vi "TX OOB Test Cases.vi"() -> (0 "error out":errorcluster, 2 "status":string, 3 "pass":bool)   [LabVIEW 2021]
uses:
  <vilib>/CIF Foundation/CIF Out of Band Commands/CIFOutOfBand.lvclass/CIFOutOfBand.ctl
  OOB_Tx/Typedef/OOB Core Commands.ctl
  typedef/Channel List for OOB.ctl
  <vilib>/CIF Foundation/CIF Channels Core/CIFChannels/Typedef/Direction.ctl
  OOB_Tx/Typedef/FIFO Publisher Return.ctl
  OOB_Tx/Private/Command Settings.vi
  <vilib>/CIF Foundation/CIF Out of Band Commands/Accessors/Write Local OOB Data.vi
  <vilib>/CIF Foundation/CIF Out of Band Commands/Queue Command.vi
  <vilib>/CIF Foundation/CIF Out of Band Commands/Utilities/Command to Bitwise Command.vi
  <vilib>/CIF Foundation/CIF Out of Band Commands/Accessors/Read Local OOB Data.vi
  <vilib>/CIF Foundation/CIF Out of Band Commands/Read Commands.vi
  OOB_Tx/Private/Read Payload.vi
  OOB_Tx/ChnMngOOB_Tx.lvclass
  C:/Program Files/National Instruments/LabVIEW 2021/vi.lib/CIF Foundation/CIF Out of Band Commands/CIFOutOfBand.lvclass
  <vilib>/CIF Foundation/CIF Out of Band Commands/Init OOB.vi
  <vilib>/CIF Foundation/CIF Out of Band Commands/CIFOutOfBand.lvclass
  <vilib>/CIF Foundation/CIF Channels Core/CIFChannels/CIFChannels.lvclass
  CIFChannelMng.lvclass
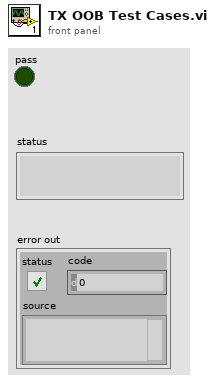
[diagram p1: front panel]
types:
  T1 = typedef "CIFChannelMng.lvclass/Channel List for OOB.ctl" = cluster{"Name":string, "Direction":T2, "Type":string, "Connected?":bool, "Connected Name":string, "Custom Config Data":u8[], "Forced?":bool}
  T2 = typedef "CIFChannels.lvclass/Direction.ctl" = enum16{"Publisher", "Subscriber"}
  T3 = typedef "ChnMngOOB_Tx.lvclass/OOB Core Commands.ctl" = enum8{"Channel List", "New FIFO Pub"}
  T4 = typedef "ChnMngOOB_Tx.lvclass/FIFO Publisher Return.ctl" = cluster{"FIFO Pub Name":string, "error":errorcluster, "Added":bool}
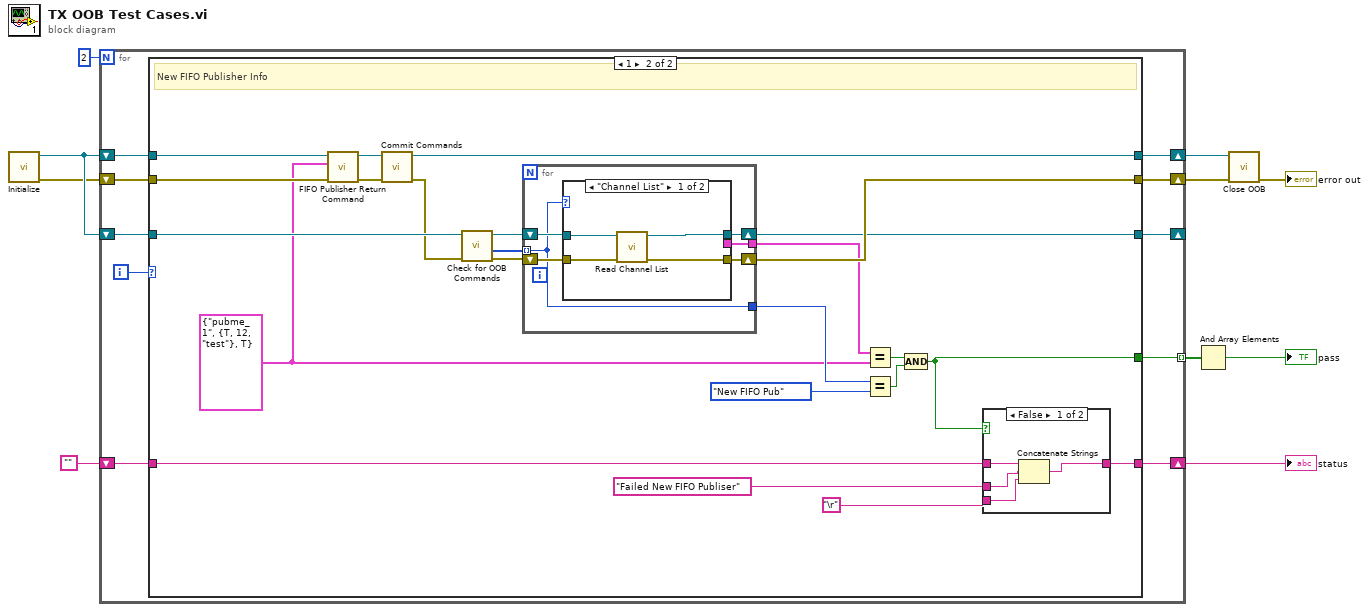
[diagram p0: block diagram]
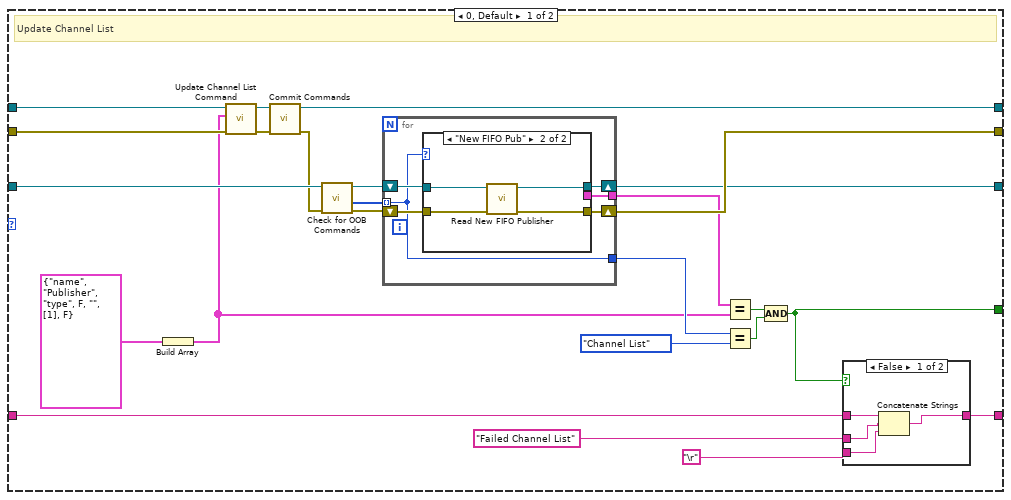
[diagram p2: hidden frame]
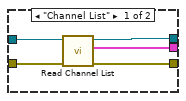
[diagram p3: hidden frame]
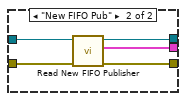
[diagram p5: hidden frame]
diagram:
  n1 = call "Initialize.vi"() -> ("error out"=w1:errorcluster, "CoreOOB_Tx out"=w2:refnum<class "ChnMngOOB_Tx.lvclass">)  [unwired: 10 in]
  n2 = for {
    N: 2 -> [_]
    tunnel: [w20] -> w8 mode=indexing
    shift-right: [w17] -> w9
    shift-left: w1 -> [w19]
    shift-right: [w12] -> w10
    shift-left: w2 -> [w18]
    shift-right: [w11] -> _
    shift-left: w2 -> [w15]
    shift-right: [w13] -> w5
    shift-left: "" -> [w14]
    i -> [w16]
    n3 = case shown="1" w16 {
      tunnel: [w36 w79] -> w20
      tunnel: w19 -> [w28 w70]
      tunnel: w18 -> [w29 w71]
      tunnel: [w44 w87] -> w17
      tunnel: [w21 w66] -> w12
      tunnel: w15 -> [w34 w77]
      tunnel: [w43 w86] -> w11
      tunnel: w14 -> [w42 w85]
      tunnel: [w41 w84] -> w13
      frame 0, Default {
        # "Update Channel List"
        n4 = Build Array(T1 {"Name"="name", "Direction"=enum."Publisher", "Type"="type", "Connected?"=FALSE, "Connected Name"="", "Custom Config Data"=[1], "Forced?"=FALSE} ("value")) -> (w25:T1[])
        n5 = call "Update Channel List Command.vi"("error in"=w28, "Channel List"=w25, "CoreOOB_Tx in"=w29) -> ("error out"=w23:errorcluster, "CoreOOB_Tx out"=w24:refnum<class "ChnMngOOB_Tx.lvclass">)  [unwired: 7 in]
        n6 = call <vilib>:"Commit Commands.vi"("error in"=w23, "OOB in"=w24) -> ("error out"=w22:errorcluster, "OOB out"=w21:refnum<class "ChnMngOOB_Tx.lvclass">)  [unwired: 8 in]
        n7 = call "Check for OOB Commands.vi"("error in (no error)"=w22, "CoreOOB_Tx in"=w34) -> ("error out"=w33:errorcluster, "Commands"=w31:T3[], "CoreOOB_Tx out"=w32:refnum<class "ChnMngOOB_Tx.lvclass">)  [unwired: 6 in, 1 out]
        n8 = for {
          tunnel: w31 -> [w46] mode=indexing
          shift-right: [w50] -> w44
          shift-left: w33 -> [w48]
          shift-right: [w49] -> w43
          shift-left: w32 -> [w47]
          tunnel: [w46] -> w35
          tunnel: [w45] -> w27
          n9 = case shown="\"New FIFO Pub\"" w46 {
            tunnel: w47 -> [w55 w59]
            tunnel: w48 -> [w54 w58]
            tunnel: [w53 w56] -> w49
            tunnel: [w52 w57] -> w50
            tunnel: [w51 _] -> w45
            frame "Channel List" {
              n10 = call "Read Channel List.vi"("error in"=w54, "CoreOOB_Tx in"=w55) -> ("error out"=w52:errorcluster, "Channel List"=w51:T1[], "CoreOOB_Tx out"=w53:refnum<class "ChnMngOOB_Tx.lvclass">)  [unwired: 7 in]
            }
            frame "New FIFO Pub" {
              n11 = call "Read New FIFO Publisher.vi"("error in"=w58, "CoreOOB_Tx in"=w59) -> ("error out"=w57:errorcluster, "CoreOOB_Tx out"=w56:refnum<class "ChnMngOOB_Tx.lvclass">)  [unwired: 7 in, 1 out]
            }
          }
        }
        n12 = Equal?(x=w27, y=w25) -> (x = y?=w38:bool)
        n13 = Equal?(x=w35, y=OOB_Core_Commands."Channel List") -> (x = y?=w37:bool)
        n14 = Compound Arithmetic op=AND(w38, w37) -> (w36:bool)
        n15 = case shown="False" w36 {
          tunnel: w42 -> [w63 w64]
          tunnel: [w60 w64] -> w41
          tunnel: "Failed Channel List" -> [w62 _]
          tunnel: "\r" -> [w61 _]
          frame False {
            n16 = Concatenate Strings(w63, w62, w61) -> (w60:string)
          }
          frame True {
          }
        }
      }
      frame 1 {
        w65 = T4 {"FIFO Pub Name"="pubme_1", "error"={"status"=TRUE, "code"=12, "source"="test"}, "Added"=TRUE} ("FIFO Publisher")
        # "New FIFO Publisher Info"
        n17 = call "FIFO Publisher Return Command.vi"("error in"=w70, "FIFO Publisher"=w65, "CoreOOB_Tx in"=w71) -> ("error out"=w68:errorcluster, "CoreOOB_Tx out"=w69:refnum<class "ChnMngOOB_Tx.lvclass">)  [unwired: 7 in]
        n18 = call <vilib>:"Commit Commands.vi"("error in"=w68, "OOB in"=w69) -> ("error out"=w67:errorcluster, "OOB out"=w66:refnum<class "ChnMngOOB_Tx.lvclass">)  [unwired: 8 in]
        n19 = call "Check for OOB Commands.vi"("error in (no error)"=w67, "CoreOOB_Tx in"=w77) -> ("error out"=w76:errorcluster, "Commands"=w74:T3[], "CoreOOB_Tx out"=w75:refnum<class "ChnMngOOB_Tx.lvclass">)  [unwired: 6 in, 1 out]
        n20 = for {
          tunnel: w74 -> [w89] mode=indexing
          shift-right: [w93] -> w87
          shift-left: w76 -> [w91]
          shift-right: [w92] -> w86
          shift-left: w75 -> [w90]
          tunnel: [w89] -> w78
          tunnel: [w88] -> w72
          n21 = case shown="\"Channel List\"" w89 {
            tunnel: w90 -> [w97 w102]
            tunnel: w91 -> [w96 w101]
            tunnel: [w95 w99] -> w92
            tunnel: [w94 w100] -> w93
            tunnel: [_ w98] -> w88
            frame "Channel List" {
              n22 = call "Read Channel List.vi"("error in"=w96, "CoreOOB_Tx in"=w97) -> ("error out"=w94:errorcluster, "CoreOOB_Tx out"=w95:refnum<class "ChnMngOOB_Tx.lvclass">)  [unwired: 7 in, 1 out]
            }
            frame "New FIFO Pub" {
              n23 = call "Read New FIFO Publisher.vi"("error in"=w101, "CoreOOB_Tx in"=w102) -> ("error out"=w100:errorcluster, "New FIFO Publisher"=w98:T4, "CoreOOB_Tx out"=w99:refnum<class "ChnMngOOB_Tx.lvclass">)  [unwired: 7 in]
            }
          }
        }
        n24 = Equal?(x=w72, y=w65) -> (x = y?=w81:bool)
        n25 = Equal?(x=w78, y=OOB_Core_Commands."New FIFO Pub") -> (x = y?=w80:bool)
        n26 = Compound Arithmetic op=AND(w81, w80) -> (w79:bool)
        n27 = case shown="False" w79 {
          tunnel: w85 -> [w106 w107]
          tunnel: [w103 w107] -> w84
          tunnel: "Failed New FIFO Publiser" -> [w105 _]
          tunnel: "\r" -> [w104 _]
          frame False {
            n28 = Concatenate Strings(w106, w105, w104) -> (w103:string)
          }
          frame True {
          }
        }
      }
    }
  }
  "status" <- w5
  n29 = And Array Elements(Boolean array=w8) -> (logical AND=→"pass":bool)
  n30 = call <vilib>:"Close OOB.vi"("error in"=w9, "OOB in"=w10) -> ("error out"=→"error out":errorcluster)  [unwired: 9 in]
